vi "SDSU_INIT.vi"(0 "Command":string, 1 "libdir":path=path "", 5 "Cmd index":i32, 7 "Cmd Option":string, 9 "Option index 2":i32, 11 "error in":errorcluster, 12 "cmdtrans":path=path "") -> (4 "ImmedReplyString":string, 15 "error out":errorcluster)   [LabVIEW 2016]
uses:
  Common/public/vis/CMN_ContStatus.ctl
  SDSU_GBLVariables.vi
  DBSHAND/private/vis/DatabaseHand_Element_Set(string).vi
  DBSHAND/private/vis/DatabaseHand_Element_Set(2DArr).vi
  DBSHAND/private/vis/DatabaseHand_Element_Set(bool).vi
  DBSHAND/private/vis/DatabaseHand_Element_Set(double).vi
panel:
  in  "AVAPP Cmd Proc":refnum<vi>
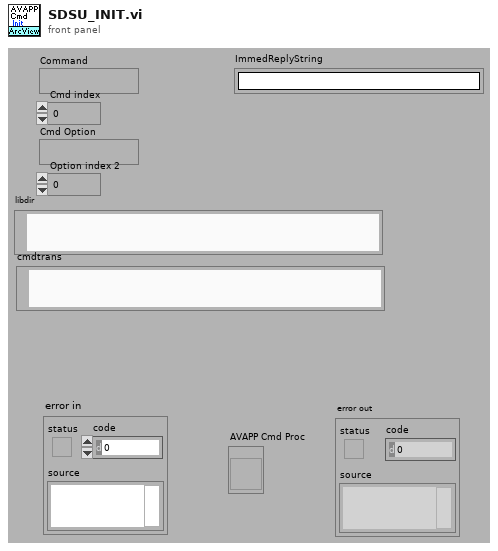
[diagram p1: front panel]
types:
  T1 = typedef "CMN_ContStatus.ctl" = cluster{"Response":string, "power":bool, "shutter":bool, "artifdata":bool, "idlemode":bool, "reset":bool, "gain":u8, "speed":u8, "resetPCI":bool, "autoshutter":bool, "TempSetPoint":i32, "multipleextensions":bool, "displayImage":bool, "coadding":bool, "images being coadded":i32, "Operation Mode":enum16{"normal", "coadd", "fawler"}, "frames to write":cluster{"subs":bool, "reset":bool, "exposed":bool}, "fawler samples":i32, "write auto":bool, "datatype":string, "frames to display":cluster{"subs":bool, "reset":bool, "exposed":bool}, "sur":i32, "autoclear":bool}
  T2 = enum16{"get fd", "set fd", "add ", "set_readtime", "get all", "clean all", "get by fd"}
  T3 = enum16{"read from file", "clear", "get all", "set all"}
  T4 = enum16{"Idle", "Exposing", "Paused", "AbortExp", "Reading", "AbortRead", "FinishedReading", "Resetting", "Reducing"}
  T5 = typedef "DatabaseHand_RefNum.ctl" = refnum<vi>
  T6 = typedef "SDSU_cmdTableEntry.ctl" = cluster{"command":string, "dsp":string, "type":string, "memtype":string, "address":i32, "bit":i32}
  T7 = typedef "DHE_Device.ctl" = cluster{"DevNo":i32, "fd":i32, "name":string, "FPA":string, "modifiers":string, "binpatt":string, "readtime":dbl, "readmode":string, "type":string, "params":string}
  T8 = cluster{"Video Processor Type":string, "support gain":bool, "Timing Board":string, "support reset":bool, "Utility Board":string, "Shutter":string, "Temperature":string, "support temp control":bool, "Detector Type":string, "Support MPP":string, "Support Binning":string, "Readout Mode":string, "support shutter control":bool}
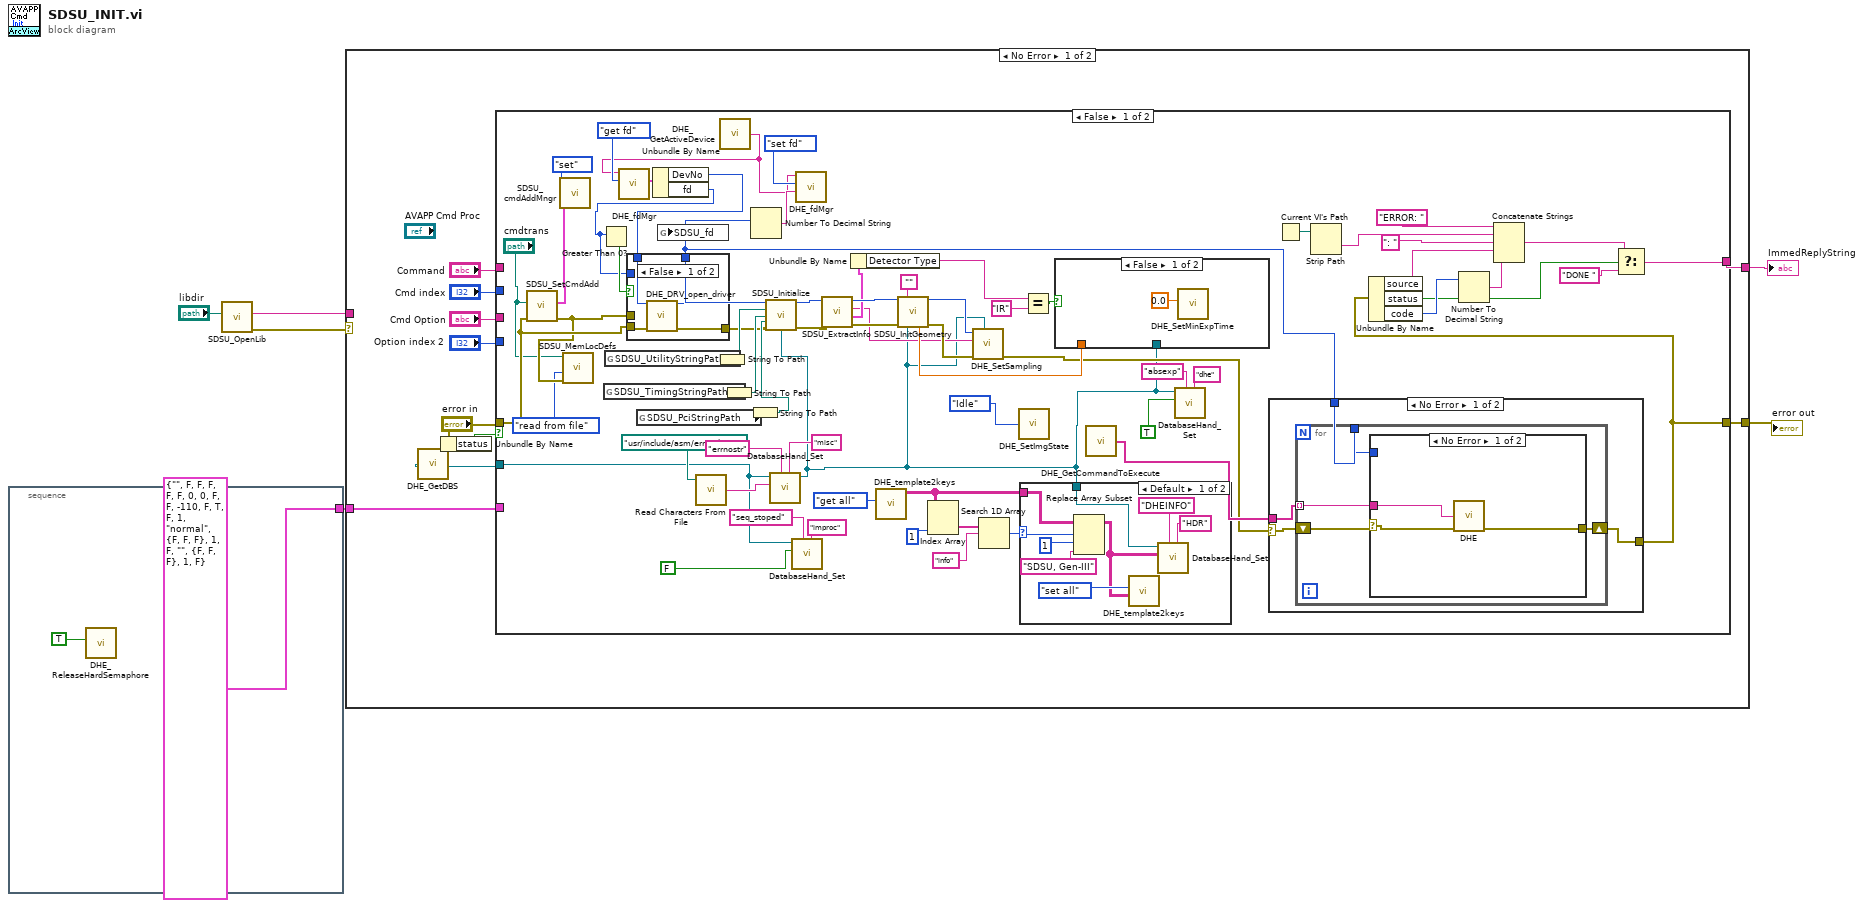
[diagram p0: block diagram]
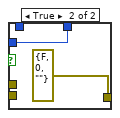
[diagram p2: hidden frame]
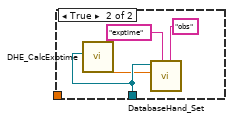
[diagram p3: hidden frame]
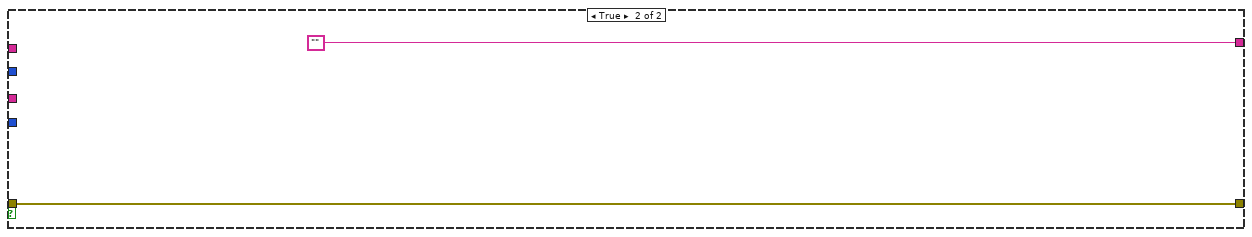
[diagram p7: hidden frame]
diagram:
  n1 = stacked-sequence {
    tunnel: [T1 {"Response"="", "power"=FALSE, "shutter"=FALSE, "artifdata"=FALSE, "idlemode"=FALSE, "reset"=FALSE, "gain"=0, "speed"=0, "resetPCI"=FALSE, "autoshutter"=FALSE, "TempSetPoint"=-110, "multipleextensions"=FALSE, "displayImage"=TRUE, "coadding"=FALSE, "images being coadded"=1, "Operation Mode"=enum."normal", "frames to write"={"subs"=FALSE, "reset"=FALSE, "exposed"=FALSE}, "fawler samples"=1, "write auto"=FALSE, "datatype"="", "frames to display"={"subs"=FALSE, "reset"=FALSE, "exposed"=FALSE}, "sur"=1, "autoclear"=FALSE} ("ControllerStatus")] -> w4
    frame #0 {
      n2 = call "DHE_ReleaseHardSemaphore.vi"("release?"=TRUE) -> ()  [unwired: 1 in, 10 out]
    }
  }
  n3 = call "SDSU_OpenLib.vi"("libdir"="libdir") -> ("error out"=w2:errorcluster, "msg out"=w1:string)  [unwired: 1 in, 8 out]
  n4 = case shown="No Error" w2 {
    selector: w2 -> [_ w123]
    tunnel: [w18 w122] -> w6
    tunnel: [w11 w123] -> w5
    tunnel: w4 -> [w10 _]
    tunnel: w1 -> [_ w122]
    frame No Error {
      n5 = call "DHE_GetDBS.vi"() -> ("DHE_DBSRef"=w9:T5)  [unwired: 9 out]
      n6 = Unbundle By Name("error in") -> ("status"=w16:bool)
      n7 = case shown="False" w16 {
        tunnel: "error in" -> [w23 w121]
        tunnel: [w68 w121] -> w11
        tunnel: [w86 ""] -> w18
        tunnel: "Command" -> [_ _]
        tunnel: "Cmd index" -> [_ _]
        tunnel: "Cmd Option" -> [_ _]
        tunnel: "Option index 2" -> [_ _]
        tunnel: w10 -> [_ _]
        tunnel: w9 -> [w40 _]
        frame False {
          n8 = call "SDSU_SetCmdAdd.vi"("error in (no error)"=w23, "translations path"="cmdtrans") -> ("error out"=w21:errorcluster, "Array"=w24:T6[])  [unwired: 8 out]
          n9 = call "SDSU_cmdAddMngr.vi"("cmds in"=w24, "action"=enum16{"find", "get", "set"}."set") -> ()  [unwired: 1 in, 9 out]
          n10 = call "SDSU_MemLocDefs.vi"("error in (no error)"=w21, "action"=enum16{"read from file", "find", "clear"}."read from file", "translations path"="cmdtrans") -> ()  [unwired: 6 in, 3 out]
          n11 = global read "SDSU_GBLVariables.vi" "SDSU_TimingStringPath"() -> (w55:string)
          n12 = global read "SDSU_GBLVariables.vi" "SDSU_UtilityStringPath"() -> (w81:string)
          n13 = global read "SDSU_GBLVariables.vi" "SDSU_PciStringPath"() -> (w67:string)
          n14 = call <vilib>:"Read Characters From File.vi"("file path (dialog if empty)"=path "/usr/include/asm/errno.h") -> ("character string"=w57:string)  [unwired: 1 in, 7 out]
          n15 = String To Path(string=w81) -> (path=w77:path)
          n16 = call "DHE_GetActiveDevice.vi"() -> ("DHE_ActiveDevice"=w30:string)  [unwired: 9 out]
          n17 = call "DHE_fdMgr.vi"("action"=T2."get fd", "cmd in"=w30) -> ("Device"=w29:T7)  [unwired: 3 in, 6 out]
          n18 = Unbundle By Name(w29) -> ("DevNo"=w27:i32, "fd"=w26:i32)
          n19 = Greater Than 0?(x=w26) -> (x > 0?=w28:bool)
          n20 = case shown="False" w28 {
            tunnel: [w90 errorcluster {"status"=FALSE, "code"=0, "source"=""} ("error out")] -> w33
            tunnel: [w89 w91] -> w32
            tunnel: w27 -> [w88 _]
            tunnel: w26 -> [_ w91]
            tunnel: w21 -> [_ _]
            tunnel: w23 -> [w87 _]
            frame False {
              n21 = call "DHE_DRV_open_driver.vi"("devno"=w88, "error in (no error)"=w87) -> ("refnum"=w89:i32, "error out"=w90:errorcluster)  [unwired: 12 out]
            }
            frame True {
            }
          }
          n22 = global write "SDSU_GBLVariables.vi" "SDSU_fd"(w32) -> ()
          n23 = String To Path(string=w55) -> (path=w76:path)
          n24 = String To Path(string=w67) -> (path=w66:path)
          n25 = Number To Decimal String(number=w32) -> (decimal integer string=w34:string)  [unwired: 1 out]
          n26 = call-poly "DatabaseHand_Set.vi"("group"="misc", "name"="errnostr", "value"=w57, "Database RefNum in"=w40) -> ("Database RefNum out"=w25:T5)  [unwired: 4 in, 3 out]
          n27 = call "SDSU_Initialize.vi"("refnum"=w32, "Utility Path"=w77, "Timing Path"=w76, "Pci Path"=w66, "error in (no error)"=w33, "Database RefNum in"=w25) -> ("refnum out"=w75:i32, "error out"=w74:errorcluster)  [unwired: 1 in, 7 out]
          n28 = call-poly "DatabaseHand_Set.vi"("group"="improc", "name"="seq_stoped" ("value"), "value"=FALSE ("Sequence was Stoped"), "Database RefNum in"=w40) -> ()  [unwired: 4 in, 4 out]
          n29 = call "DHE_fdMgr.vi"("arg in"=w34, "action"=T2."set fd", "cmd in"=w30) -> ()  [unwired: 2 in, 7 out]
          n30 = call "SDSU_ExtractInfo.vi"("error in (no error)"=w74, "refnum"=w75) -> ("error out"=w73:errorcluster, "ControllerConfigCluster"=w54:T8, "Detector Type"=w37:string, "refnum out"=w72:i32)  [unwired: 6 out]
          n31 = Unbundle By Name(w54) -> ("Detector Type"=w53:string)
          n32 = call "DHE_template2keys.vi"("Action"=T3."get all") -> ("HdrInfo"=w60:string[][])  [unwired: 3 in, 7 out]
          n33 = call "SDSU_InitGeometry.vi"("refnum"=w72, "override format"="", "error in (no error)"=w73, "Database RefNum out"=w25) -> ("fd out"=w36:i32, "DET_READ_TIME"=w50:sgl, "error out"=w38:errorcluster)  [unwired: 9 out]
          n34 = Index Array(array=w60, index (col)=1 ("index (row)")) -> (element=w63:string[])  [unwired: 1 in]
          n35 = call "DHE_SetSampling.vi"("DBS Ref"=w25, "error in"=w38, "sampling type"=w37, "fd"=w36) -> ("error out"=w39:errorcluster)  [unwired: 7 out]
          n36 = Search 1D Array(1D array=w63, element="info") -> (index of element=w61:i32)  [unwired: 1 out]
          n37 = call "DHE_SetImgState.vi"("DHE_ImgState"=T4."Idle" ("ImgState")) -> ()  [unwired: 9 out]
          n38 = case shown="Default" w61 {
            selector: w61 -> [w104 _]
            tunnel: w60 -> [w105 _]
            tunnel: w25 -> [w98 _]
            frame Default {
              n39 = Replace Array Subset(array=w105, new element="SDSU, Gen-III" ("new element/subarray"), index (row)=w104, index (col)=1 ("disabled index (col)")) -> (w99:string[][])
              n40 = call "DHE_template2keys.vi"("HdrInfo In"=w99, "Action"=T3."set all") -> ()  [unwired: 2 in, 8 out]
              n41 = call-poly "DatabaseHand_Set.vi"("group"="HDR", "name"="DHEINFO", "value"=w99, "Database RefNum in"=w98) -> ()  [unwired: 4 in, 4 out]
            }
            frame ..-1 {
            }
          }
          n42 = Equal?(x=w53, y="IR") -> (x = y?=w51:bool)
          n43 = case shown="False" w51 {
            tunnel: w50 -> [_ _]
            tunnel: w25 -> [_ w95]
            frame False {
              n44 = call "DHE_SetMinExpTime.vi"("MinExpTime"=sgl 0.0) -> ()  [unwired: 11 out]
            }
            frame True {
              n45 = call "DHE_CalcExptime.vi"("DHE_DBSRef"=w95) -> ("min_exp_time"=w94:dbl)  [unwired: 1 in, 9 out]
              n46 = call-poly "DatabaseHand_Set.vi"("group"="obs", "name"="exptime", "value"=w94, "Database RefNum in"=w95) -> ()  [unwired: 4 in, 4 out]
            }
          }
          n47 = call "DHE_GetCommandToExecute.vi"() -> ("DHE_Commands2Exec"=w41:string[])  [unwired: 9 out]
          n48 = call-poly "DatabaseHand_Set.vi"("group"="dhe", "name"="absexp", "value"=TRUE, "Database RefNum in"=w25) -> ()  [unwired: 4 in, 4 out]
          n49 = case shown="No Error" w39 {
            selector: w39 -> [w107 w119]
            tunnel: w41 -> [w110 _]
            tunnel: [w109 w119] -> w68
            tunnel: w32 -> [w108 _]
            frame No Error {
              n50 = for {
                tunnel: w108 -> [w114]
                tunnel: w110 -> [w111] mode=indexing
                shift-right: [w112] -> w109
                shift-left: w107 -> [w113]
                n51 = case shown="No Error" w113 {
                  selector: w113 -> [w117 w118]
                  tunnel: w114 -> [_ _]
                  tunnel: [w116 w118] -> w112
                  tunnel: w111 -> [w115 _]
                  frame No Error {
                    n52 = call "DHE.vi"("Cmd"=w115, "error in"=w117) -> ("error out"=w116:errorcluster)  [unwired: 1 in, 12 out]
                  }
                  frame Error {
                  }
                }
              }
            }
            frame Error {
            }
          }
          n53 = Current VI's Path() -> (path=w85:path)
          n54 = Strip Path(path=w85) -> (name=w80:string)  [unwired: 1 out]
          n55 = Unbundle By Name(w68) -> ("source"=w69:string, "status"=w70:bool, "code"=w71:i32)
          n56 = Number To Decimal String(number=w71) -> (decimal integer string=w78:string)  [unwired: 1 out]
          n57 = Concatenate Strings("ERROR: ", w80, ": ", w69, w78) -> (w83:string)
          n58 = Select(t=w83, s=w70, f="DONE ") -> (s? t:f=w86:string)
        }
        frame True {
        }
      }
    }
    frame Error {
    }
  }
  "error out" <- w5
  "ImmedReplyString" <- w6
